vi "DFT_Spectra UI.vi"(10 "averages completed":dbl, 11 "Spectrum Data":refnum<class "Data.lvclass">) -> ()   [LabVIEW 2023, in "DFT_Spectra.lvlib" / "DFT_Spectra.lvclass"]
uses:
  DFT_Spectra.lvclass
  <vilib>/addons/_XControls/Spectrum with Cursors/Spectrum with Cursors.xctl
  <vilib>/addons/_NISVFA/_Shared subVIs/Data Objects/Data/Data.lvclass
panel:
  out "Averages completed":dbl
  out "Spectrum with Cursors":refnum<class "Data.lvclass">(xcontrol)
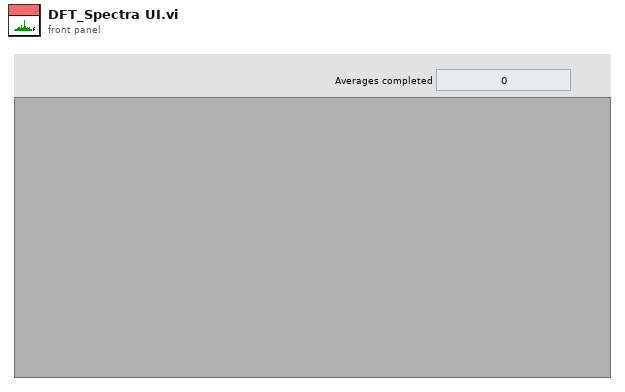
[diagram p1: front panel]
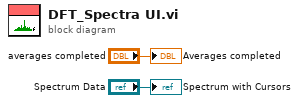
[diagram p0: block diagram]
diagram:
  "Averages completed" <- "averages completed"
  "Spectrum with Cursors" <- "Spectrum Data"
